vi "CALL_WT333E.vi"(11 "simulazione":bool) -> ()   [LabVIEW 2019]
panel:
  out "Iteration":i32
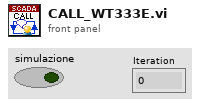
[diagram p1: front panel]
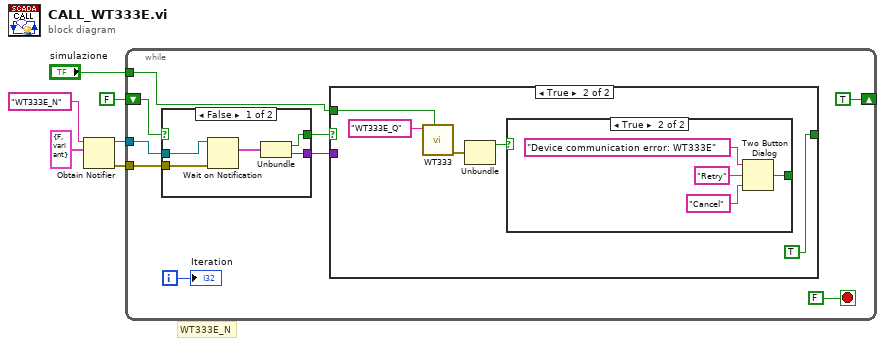
[diagram p0: block diagram]
diagram:
  # "WT333E_N"
  n1 = Obtain Notifier(name (unnamed)="WT333E_N" ("Notifier Name"), notification data type=cluster{"boolean":bool, "variant":variant} {"boolean"=FALSE, "variant"=variant} ("notification")) -> (notifier out=w4:refnum<notifier>, error out=w5:errorcluster)  [unwired: 2 in, 1 out]
  n2 = while {
    tunnel: "simulazione" -> [w15]
    tunnel: w5 -> [w13]
    tunnel: w4 -> [w14]
    shift-right: [TRUE] -> _
    shift-left: FALSE -> [w11]
    i -> [w9]
    stop <- FALSE stop-if-true
    n3 = case shown="False" w11 {
      selector: w11 -> [_ w21]
      tunnel: w14 -> [w20 _]
      tunnel: w13 -> [w19 _]
      tunnel: [w17 w21] -> w8
      tunnel: [w16 _] -> w12
      frame False {
        n4 = Wait on Notification(notifier=w20, error in (no error)=w19) -> (notification=w18:cluster{"boolean":bool, "variant":variant})  [unwired: 2 in, 3 out]
        n5 = Unbundle(w18) -> ("boolean"=w17:bool, "variant"=w16:variant)
      }
      frame True {
      }
    }
    n6 = case shown="True" w8 {
      selector: w8 -> [w22 _]
      tunnel: [w22 TRUE] -> _
      tunnel: w12 -> [_ _]
      tunnel: w15 -> [_ w26]
      frame False {
      }
      frame True {
        n7 = call "WT333.vi"("simulazione"=w26, "Queue Name"="WT333E_Q") -> ("error out"=w27:errorcluster)  [unwired: 8 in, 1 out]
        n8 = Unbundle(w27) -> ("status"=w24:bool)  [unwired: 2 out]
        n9 = case shown="True" w24 {
          tunnel: [_ w28] -> _
          frame False {
          }
          frame True {
            n10 = Two Button Dialog(message="Device communication error: WT333E", 1:"Cancel" ("Right Button Text (\"Cancel\")"), 2:"Retry" ("Left Button Text (\"Yes\")")) -> (T button?=w28:bool)
          }
        }
      }
    }
    "Iteration" <- w9
  }
